vi "Master, Append Step Name.vi"(4 "Enable (T)":bool=TRUE, 5 "step name":string="Sequence Step General: Name", 6 "error in":errorcluster, 8 "BGColor (Orange)":u32(colorbox)=16635906, 9 "Tbl Refnum":refnum<vi>) -> (0 "error out":errorcluster, 2 "row_n (I32)":i32=-1, 3 "Tbl Refnum dup":refnum<vi>)   [LabVIEW 2010]
doc: "This function appends a step name to a table in column one (zero index), sets the cell background color, and sets the cell font to bold."
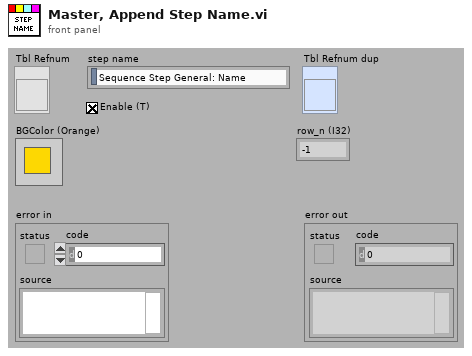
[diagram p1: front panel]
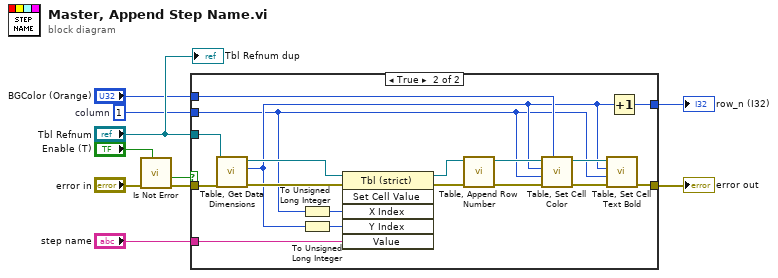
[diagram p0: block diagram]
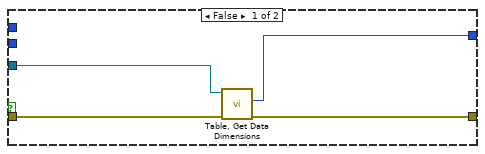
[diagram p2: hidden frame]
diagram:
  w6 = 1  # column
  n1 = call "Is Not Error.vi"("enable (T)"="Enable (T)", "error in"="error in") -> ("error out"=w3:errorcluster, "ready"=w2:bool)  [unwired: 4 in, 1 out]
  n2 = case shown="True" w2 {
    tunnel: "Tbl Refnum" -> [w11 w32]
    tunnel: [w13 w19] -> w9
    tunnel: [w12 w27] -> w8
    tunnel: "step name" -> [_ w30]
    tunnel: w6 -> [_ w16]
    tunnel: "BGColor (Orange)" -> [_ w25]
    tunnel: w3 -> [w14 w15]
    frame False {
      n3 = call "Table, Get Data Dimensions.vi"("error in"=w14, "Tbl Refnum"=w11) -> ("error out"=w13:errorcluster, "row_n"=w12:i32)  [unwired: 6 in, 2 out]
    }
    frame True {
      n4 = call "Table, Get Data Dimensions.vi"("error in"=w15, "Tbl Refnum"=w32) -> ("error out"=w31:errorcluster, "row_n"=w17:i32, "Tbl Refnum out"=w28:refnum<vi>)  [unwired: 6 in, 1 out]
      n5 = To Unsigned Long Integer(number=w16) -> (unsigned 32bit integer=w26:u32)
      n6 = To Unsigned Long Integer(number=w17) -> (unsigned 32bit integer=w29:u32)
      n7 = invoke class="Tbl (strict)" method="Set Cell Value"(reference=w28, error in=w31, "X Index"=w26, "Y Index"=w29, "Value"=w30) -> (reference out=w23:refnum<vi>, error out=w24:errorcluster)  [unwired: 1 in, 4 out]
      n8 = call "Table, Append Row Number.vi"("error in"=w24, "Tbl Refnum"=w23) -> ("error out"=w22:errorcluster, "Tbl Refnum out"=w21:refnum<vi>)  [unwired: 8 in]
      n9 = call "Table, Set Cell Color.vi"("BGColor Enabled"=w25, "error in"=w22, "col (0)"=w16, "row (0)"=w17, "Tbl Refnum"=w21) -> ("error out"=w20:errorcluster, "Tbl Refnum out"=w18:refnum<vi>)  [unwired: 2 in, 2 out]
      n10 = call "Table, Set Cell Text Bold.vi"("error in"=w20, "col (0)"=w16, "row (0)"=w17, "Tbl Refnum"=w18) -> ("error out"=w19:errorcluster)  [unwired: 2 in, 3 out]
      n11 = Increment(x=w17) -> (x+1=w27:i32)
    }
  }
  "row_n (I32)" <- w8
  "error out" <- w9
  "Tbl Refnum dup" <- "Tbl Refnum"
